vi "checkNode.vi"(2 "PubSub":T1, 3 "ROS_Master":refnum<class "ROS_Master.lvclass">) -> (1 "ROS_Master out":refnum<class "ROS_Master.lvclass">)   [LabVIEW 2012, in "ROS_Master.lvclass"]
doc: "Checks to see if the node for this topic has already been specified. If it has, but with a different IP, the master will send a shutdown message to the old node and update the node to the new address. Else, adds the new node to the list."
uses:
  ROS_Master.lvclass
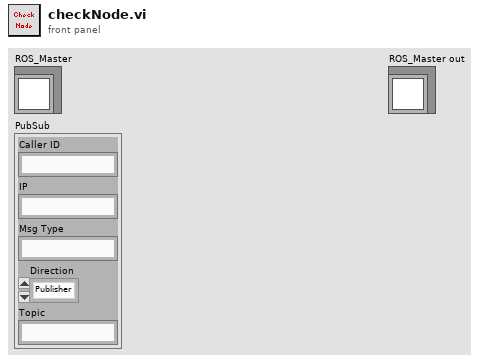
[diagram p1: front panel]
types:
  T1 = cluster{"Caller ID":string, "IP":string, "Msg Type":string, "Direction":enum16{"Publisher", "Subscriber"}, "Topic":string}
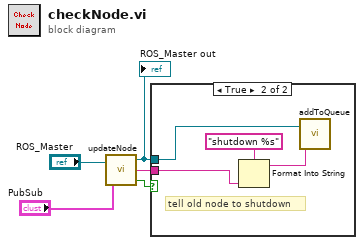
[diagram p0: block diagram]
diagram:
  n1 = call "updateNode.vi"("ROS_Master in"="ROS_Master", "PubSub in"="PubSub") -> ("ROS_Master out"=w3:refnum<class "ROS_Master.lvclass">, "Shutdown URI"=w4:string, "shutdown needed?"=w1:bool)
  "ROS_Master out" <- w3
  n2 = case shown="True" w1 {
    tunnel: w4 -> [_ w6]
    tunnel: w3 -> [_ w7]
    frame False {
    }
    frame True {
      # "tell old node to shutdown"
      n3 = Format Into String(format string="shutdown %s", w6) -> (resulting string=w8:string)  [unwired: 2 in, 1 out]
      n4 = call "addToQueue.vi"("Message"=w8, "ROS_Master"=w7) -> ()  [unwired: 2 in]
    }
  }
